vi "Step7_0_LowPass.vi"(9 "s_axis_data_tdata":fxp<+/-,24,1>, 10 "s_axis_data_tvalid":bool) -> (1 "m_axis_data_tdata":fxp<+/-,24,2>, 2 "m_axis_data_tvalid":bool, 3 "s_axis_data_tready":bool)   [LabVIEW 2018]
uses:
  <vilib>/rvi/IPIntegrationNode/IPINode_Typedef/niFpgaIPINodeSupportedFamilies.ctl
  <vilib>/rvi/IPIntegrationNode/IPINode_Utilities/niFpgaIPINodeSimCore.vi
  <vilib>/rvi/XilinxIP/XIPIN_XNode/niFpgaXIPIN.xnode
  FIR_Filter_Configuration/FIR Compiler/xsim.dir/FIR_Compiler_3CE652926F5B43F18022D1349C670FA0/xsimk_3CE652926F5B43F18022D1349C670FA0.dll
  <vilib>/rvi/IPIntegrationNode/IPINode_Xnode/niFpgaIPINode.xnode
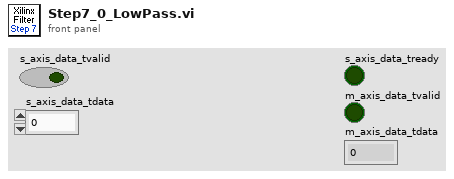
[diagram p1: front panel]
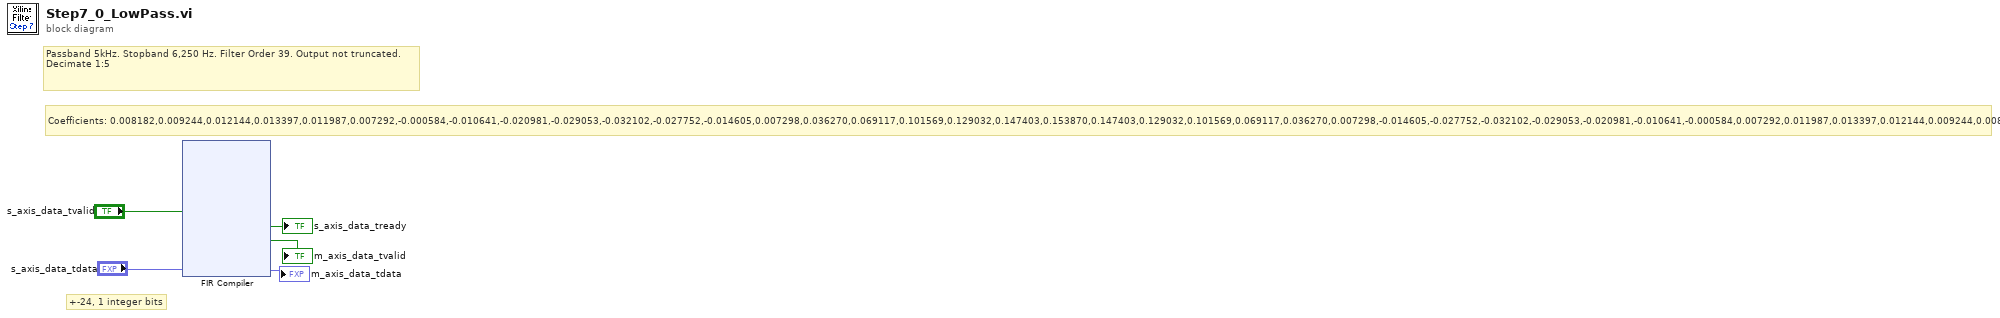
[diagram p0: block diagram]
diagram:
  # "+-24, 1 integer bits"
  # "Coefficients: 0.008182,0.009244,0.012144,0.013397,0.011987,0.007292,-0.000584,-0.010641,-0.020981,-0.029053,-0.032102,-0.027752,-0.014605,0.007298,0.036270,0.069117,0.101569,0.129032,0.147403,0.153870,0.147403,0.129032,0.101569,0.069117,0.036270,0.007298,-0.014605,-0.027752,-0.032102,-0.029053,-0.020981,-0.010641,-0.000584,0.007292,0.011987,0.013397,0.012144,0.009244,0.008182"
  # "Passband 5kHz. Stopband 6,250 Hz. Filter Order 39. Output not truncated.\nDecimate 1:5"
  n1 = xnode ("FIR Compiler")("s_axis_data_tvalid"="s_axis_data_tvalid", "s_axis_data_tdata"="s_axis_data_tdata") -> ("s_axis_data_tready"=→"s_axis_data_tready":bool, "m_axis_data_tvalid"=→"m_axis_data_tvalid":bool, "m_axis_data_tdata"=→"m_axis_data_tdata":fxp<+/-,24,2>)
